vi "two string adding 6.vi"() -> ()   [LabVIEW 2025]
panel:
  out "o/p":string
  in  "s2":string
  in  "s1":string
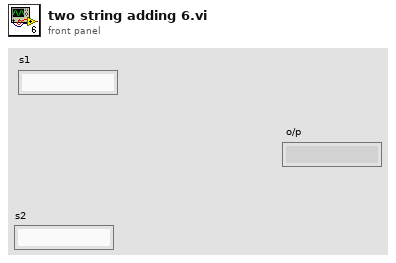
[diagram p1: front panel]
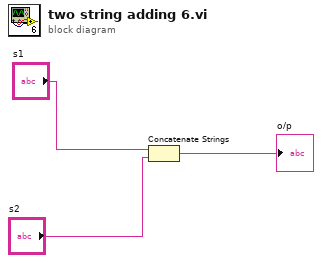
[diagram p0: block diagram]
diagram:
  n1 = Concatenate Strings("s1", "s2") -> (→"o/p":string)
